vi "Actor Core.vi"(8 "error in":errorcluster, 11 "Measure Object in":refnum<class "Micron Optics Recorder.lvclass">) -> (0 "error out":errorcluster, 3 "Actor out":refnum<class "Actor.lvclass">)   [LabVIEW 2016, in "Micron Optics Recorder.lvclass"]
doc: "(<B>Filename</B>: Actor Framework.lvlib:Actor.lvclass:Actor Core.vi)\n\nReceives messages to the actor, reacts to them, and initiates any error handling that may shut the actor down.\n\nDescendant classes may override this VI to append parallel tasks for the actor to complete while it handles messages. Overrides use the Call Parent Method node."
uses:
  Micron Optics Recorder.lvclass
  Instrument Actor/Instrument Actor.lvclass
  <vilib>/ActorFramework/Actor/Actor.lvclass
  Micron Optics Recorder Messages/Plot Spectrum Msg/Plot Spectrum Msg.lvclass
  C:/Program Files (x86)/National Instruments/LabVIEW 2016/vi.lib/ActorFramework/Actor/Actor.lvclass
  NHMFL_Core/Libraries/Instruments/Micron Optics/Micron optics configuration.ctl
panel:
  in  "Configuration":T1={"Reference channel"=-1, "Detection Setting IDs"=[130, 130], "Address"="192.168.1.55", "Stream and average"=TRUE}
  out "Name":string
  in  "Refresh  specrum":bool
  out "Spectrum Graph":cluster{dbl[], "Spectrum, db":dbl[]}[](graph)
  # "CH1\n.\n.\n.\n.\n.\nCH4"
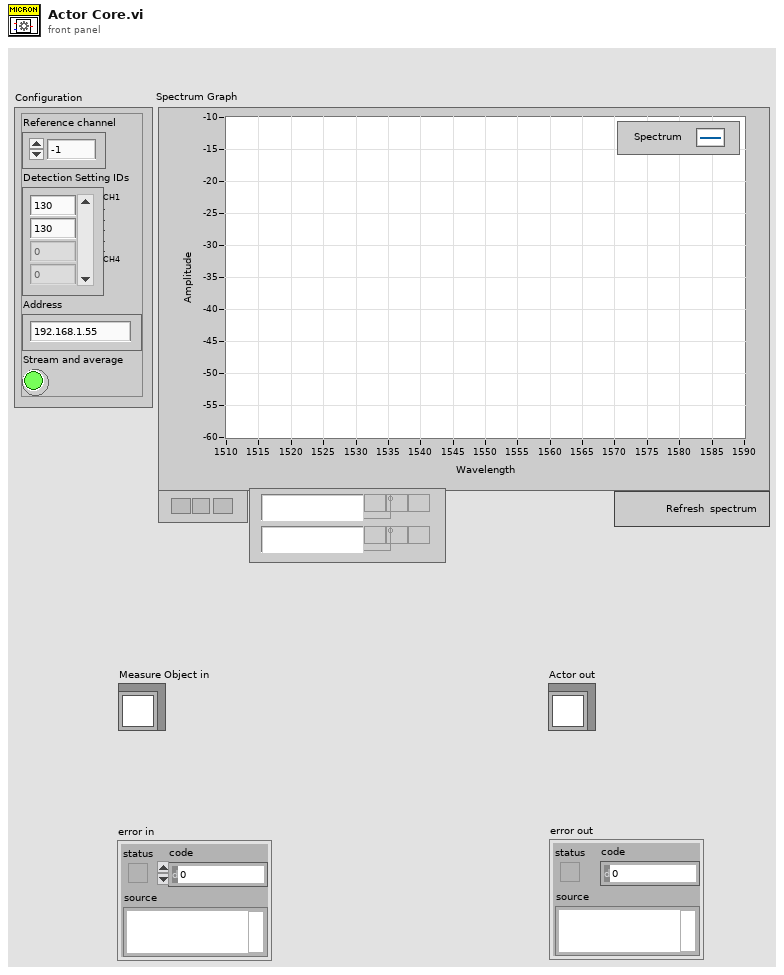
[diagram p1: front panel]
types:
  T1 = typedef "Micron optics configuration.ctl" = cluster{"Reference channel":i32, "Detection Setting IDs":u8[], "Address":string, "Stream and average":bool}
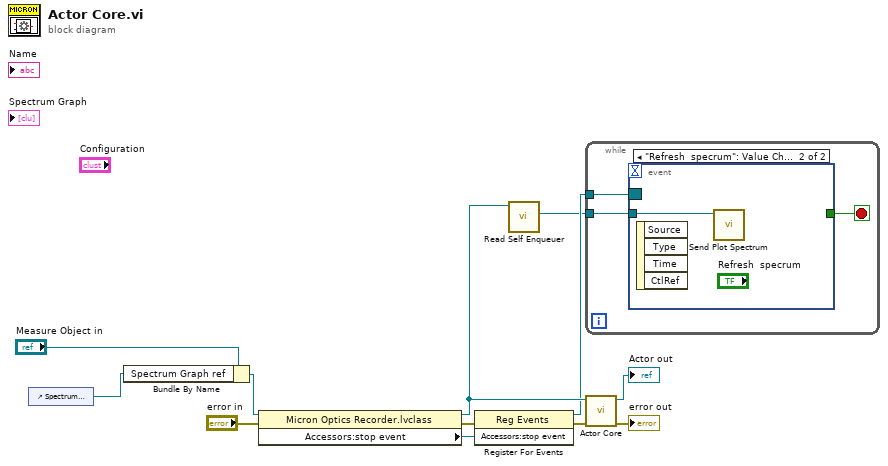
[diagram p0: block diagram]
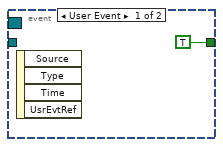
[diagram p2: hidden frame]
diagram:
  n1 = control-ref of="Spectrum Graph"() -> (w2:refnum<vi>)
  n2 = Bundle By Name(cluster="Measure Object in", "Spectrum Graph ref"=w2) -> (w3:refnum<class "Micron Optics Recorder.lvclass">)
  n3 = property class="Micron Optics Recorder.lvclass"(reference=w3, error in="error in") -> (reference out=w5:refnum<class "Micron Optics Recorder.lvclass">, error out=w9:errorcluster, "Accessors:stop event"=w10:refnum<user-event>)
  n4 = register-events(error in=w9, w10) -> (reference out=w4:refnum<event-registration>, error out=w6:errorcluster)  [unwired: 1 in]
  n5 = call <vilib>:"Read Self Enqueuer.vi"("Actor"=w5) -> ("Self Enqueuer"=w1:refnum<class "Message Enqueuer.lvclass">)  [unwired: 10 in]
  n6 = while {
    tunnel: w4 -> [w15]
    tunnel: w1 -> [w13]
    stop <- w14 stop-if-true
    n7 = event shown="[1] \"Refresh  specrum\": Value Change" {
      selector: w15 -> [_ _]
      dyn-events: _ -> [_ _]
      timeout: _ -> [_ _]
      tunnel: [TRUE _] -> w14
      tunnel: w13 -> [_ w17]
      event User Event {
        n8 = event-data() -> ()  [unwired: 1 in, 4 out]
      }
      event "Refresh  specrum": Value Change {
        n9 = event-data() -> ()  [unwired: 1 in, 4 out]
        n10 = call "Send Plot Spectrum.vi"("Message Enqueuer"=w17) -> ()  [unwired: 9 in, 2 out]
      }
    }
  }
  n11 = call-parent "Actor Core.vi"("error in"=w6, "Measure Object in"=w5) -> ("error out"=→"error out":errorcluster, "Actor out"=→"Actor out":refnum<class "Actor.lvclass">)  [unwired: 8 in]
